vi "Mixer.Initialize.vi"(1 "baseURL":string="169.254.221.196") -> ()   [LabVIEW 2020]
panel:
  # "http://169.254.221.196/"
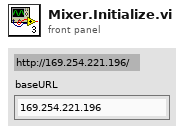
[diagram p1: front panel]
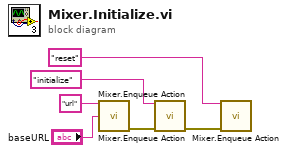
[diagram p0: block diagram]
diagram:
  n1 = call "Mixer.Enqueue Action.vi"("action"="url", "data"="baseURL") -> ("error out"=w4:errorcluster)  [unwired: 13 in]
  n2 = call "Mixer.Enqueue Action.vi"("action"="initialize", "error in (no error)"=w4) -> ("error out"=w1:errorcluster)  [unwired: 13 in]
  n3 = call "Mixer.Enqueue Action.vi"("action"="reset", "error in (no error)"=w1) -> ()  [unwired: 13 in, 1 out]
